vi "retrieve control values.vi"(8 "error in (no error)":errorcluster, 11 "path":path) -> (0 "error out":errorcluster, 3 "path out":path)   [LabVIEW 2020, in "POLARIS Vision utility.lvlib"]
doc: "from ni.com \nauthor mmiers."
uses:
  POLARIS Vision utility.lvlib
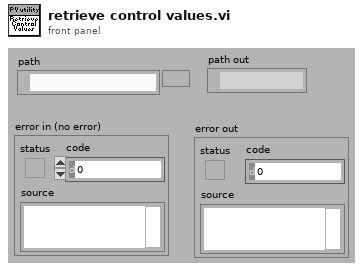
[diagram p1: front panel]
types:
  T1 = enum32{"invalid app kind", "Development System", "Run Time System", "Student Edition", "Embedded LabVIEW", "Evaluation", "Custom"}
  T2 = cluster{"Name":string, "type string":i16[], "data string":string}[]
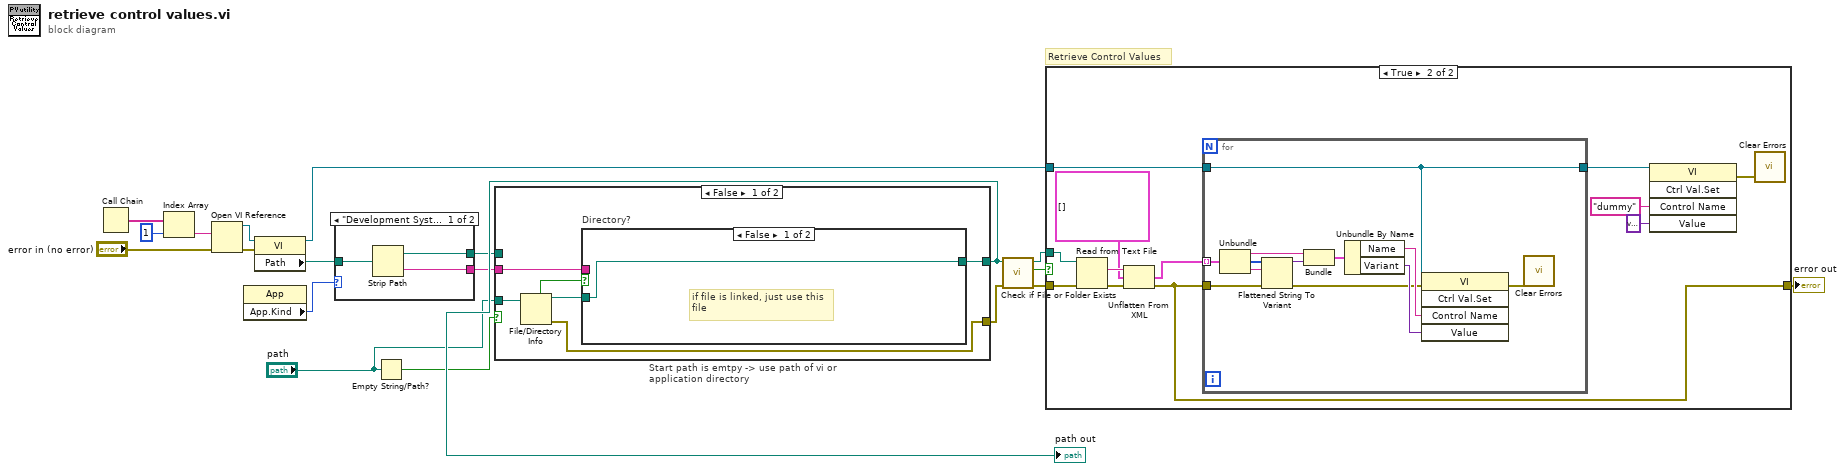
[diagram p0: block diagram]
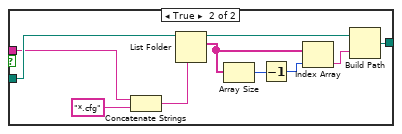
[diagram p2: hidden frame]
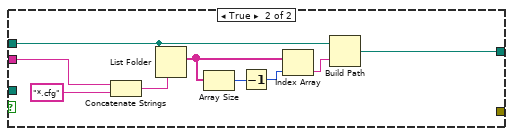
[diagram p3: hidden frame]
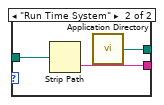
[diagram p4: hidden frame]
diagram:
  # "Retrieve Control Values"
  n1 = Call Chain() -> (call chain=w19:string[])
  n2 = Index Array(array=w19, index=1) -> (element=w11:string)
  n3 = Open VI Reference(vi path=w11, error in (no error)="error in (no error)") -> (vi reference=w10:refnum<vi>, error out=w14:errorcluster)  [unwired: 4 in]
  n4 = property class="App"() -> ("App.Kind"=w7:T1)  [unwired: 2 in, 2 out]
  n5 = property class="VI"(reference=w10, error in=w14) -> (reference out=w6:refnum<vi>, "Path"=w8:path)  [unwired: 1 out]
  n6 = case shown="\"Development System\", Default" w7 {
    tunnel: w8 -> [w21 w24]
    tunnel: [w22 w23] -> w5
    tunnel: [w20 w25] -> w4
    frame "Development System", Default {
      n7 = Strip Path(path=w21) -> (stripped path=w22:path, name=w20:string)
    }
    frame "Run Time System" {
      n8 = Strip Path(path=w24) -> (name=w25:string)  [unwired: 1 out]
      n9 = call <vilib>:"Application Directory.vi"() -> ("Application Directory"=w23:path)
    }
  }
  n10 = Empty String/Path?(string/path="path") -> (empty?=w3:bool)
  n11 = case "Start path is emtpy -> use path of vi or application directory" shown="False" w3 {
    tunnel: [w28 w51] -> w9
    tunnel: w5 -> [_ w44]
    tunnel: w4 -> [w27 w43]
    tunnel: "path" -> [w31 _]
    tunnel: [w26 _] -> w1
    frame False {
      n12 = File/Directory Info(path=w31) -> (path out=w29:path, directory=w30:bool, error out=w26:errorcluster)  [unwired: 1 in, 4 out]
      n13 = case "Directory?" shown="False" w30 {
        tunnel: w29 -> [w32 w36]
        tunnel: [w32 w34] -> w28
        tunnel: w27 -> [_ w33]
        frame False {
          # "if file is linked, just use this\nfile"
        }
        frame True {
          n14 = Concatenate Strings(w33, "*.cfg" ("string")) -> (w42:string)
          n15 = List Folder(path=w36, pattern=w42) -> (path out=w35:path, filenames=w40:string[])  [unwired: 2 in, 2 out]
          n16 = Array Size(array=w40) -> (size(s)=w39:i32)
          n17 = Decrement(x=w39) -> (x-1=w38:i32)
          n18 = Index Array(array=w40, index=w38) -> (element=w37:string)
          n19 = Build Path(base path=w35, name or relative path=w37) -> (appended path=w34:path)
        }
      }
    }
    frame True {
      n20 = Concatenate Strings(w43, "*.cfg" ("string")) -> (w50:string)
      n21 = List Folder(path=w44, pattern=w50) -> (filenames=w48:string[])  [unwired: 2 in, 3 out]
      n22 = Array Size(array=w48) -> (size(s)=w47:i32)
      n23 = Decrement(x=w47) -> (x-1=w46:i32)
      n24 = Index Array(array=w48, index=w46) -> (element=w45:string)
      n25 = Build Path(base path=w44, name or relative path=w45) -> (appended path=w51:path)
    }
  }
  "path out" <- w9
  n26 = call <vilib>:"Check if File or Folder Exists.vi"("error in (no error)"=w1, "path"=w9) -> ("error out"=w13:errorcluster, "file or folder exists?"=w16:bool, "dup path"=w17:path)  [unwired: 7 in]
  n27 = case shown="True" w16 {
    tunnel: w6 -> [_ w60]
    tunnel: w17 -> [_ w59]
    tunnel: w13 -> [w52 w58]
    tunnel: [w52 w53] -> w12
    frame False {
    }
    frame True {
      n28 = Read from Text File(file (use dialog)=w59, error in=w58) -> (text=w64:string, error out=w63:errorcluster)  [unwired: 4 out]
      n29 = Unflatten From XML(xml string=w64, type=T2 [], error in (no error)=w63) -> (value=w61:T2, error out=w53:errorcluster)
      n30 = for {
        tunnel: w53 -> [w75]
        tunnel: w61 -> [w72] mode=indexing
        tunnel: w60 -> [w66]
        tunnel: [w66] -> w57
        n31 = Unbundle(w72) -> ("Name"=w73:string, "type string"=w71:i16[], "data string"=w70:string)
        n32 = Flattened String To Variant(4:w75, 6:w70, 7:w71) -> (0:w67:errorcluster, 3:w74:variant)
        n33 = Bundle("Name"=w73, "Variant"=w74) -> (w69:cluster{"Name":string, "Variant":variant})  [unwired: 1 out]
        n34 = Unbundle By Name(w69) -> ("Name"=w68:string, "Variant"=w76:variant)
        n35 = invoke class="VI" method="Ctrl Val.Set"(reference=w66, error in=w67, "Control Name"=w68, "Value"=w76) -> (error out=w65:errorcluster)  [unwired: 1 in, 4 out]
        n36 = call <vilib>:"Clear Errors.vi"("error in (no error)"=w65) -> ()  [unwired: 5 in, 2 out]
      }
      n37 = invoke class="VI" method="Ctrl Val.Set"(reference=w57, "Control Name"="dummy", "Value"=variant) -> (error out=w54:errorcluster)  [unwired: 2 in, 4 out]
      n38 = call <vilib>:"Clear Errors.vi"("error in (no error)"=w54) -> ()  [unwired: 5 in, 2 out]
    }
  }
  "error out" <- w12
